vi "AHRead2550.vi"(8 "error in (no error)":errorcluster) -> (0 "error out":errorcluster, 2 "loss":dbl=nan format="%.7f", 3 "capacitance":dbl=nan format="%.7f")   [LabVIEW 2009]
uses:
  <instrlib>/Andeen-Hagerling 2550/Andeen-Hagerling 2550.lvlib
panel:
  out "Loss Chart":dbl(graph)
  out "Cap Chart":dbl(graph)
  out "Vexc":dbl=nan format="%.7f"
  out "out string":string
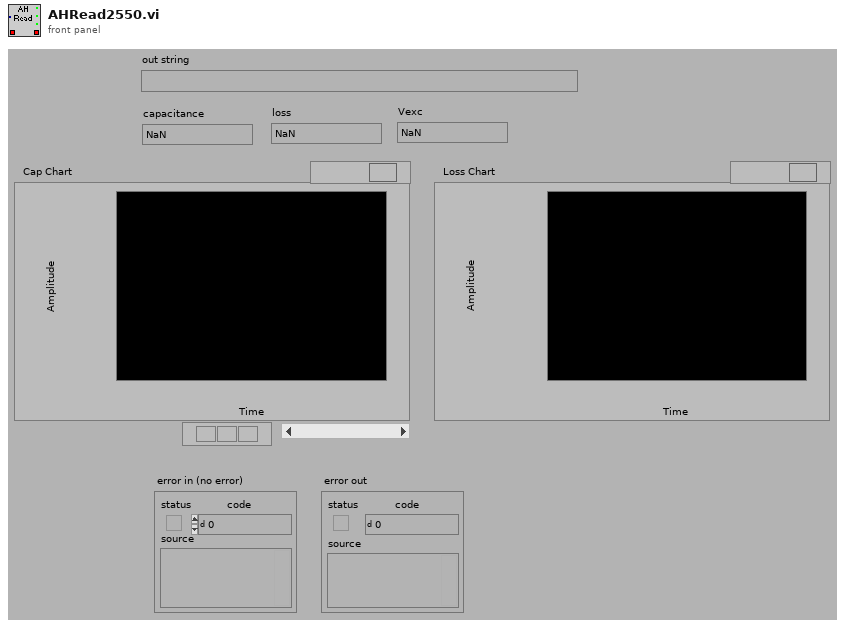
[diagram p1: front panel]
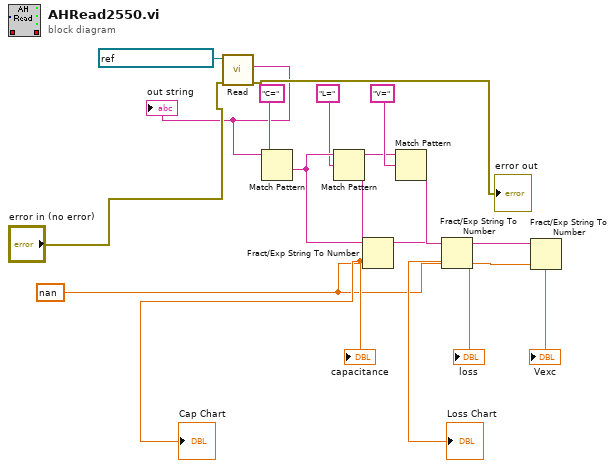
[diagram p0: block diagram]
diagram:
  w5 = nan ("default (0 dbl)")
  n1 = call <instrlib>:"Read.vi"("error in"="error in (no error)", "VISA resource name"=refnum<visa-resource-name> "GPIB0::28::INSTR") -> ("error out"=→"error out":errorcluster, "Message"=w1:string)  [unwired: 6 in, 2 out]
  "out string" <- w1
  n2 = Match Pattern(string=w1, regular expression="C=") -> (after substring=w13:string)  [unwired: 1 in, 3 out]
  n3 = Match Pattern(string=w13, regular expression="L=") -> (after substring=w9:string)  [unwired: 1 in, 3 out]
  n4 = Fract/Exp String To Number(string=w13, default (0 dbl)=w5) -> (number=→"capacitance" →"Cap Chart":dbl)  [unwired: 2 in, 1 out]
  n5 = Match Pattern(string=w9, regular expression="V=") -> (after substring=w11:string)  [unwired: 1 in, 3 out]
  n6 = Fract/Exp String To Number(string=w9, default (0 dbl)=w5) -> (number=→"loss" →"Loss Chart":dbl)  [unwired: 2 in, 1 out]
  n7 = Fract/Exp String To Number(string=w11, default (0 dbl)=w5) -> (number=→"Vexc":dbl)  [unwired: 2 in, 1 out]
